vi "lvBuildAll.vi"() -> (0 "error out":errorcluster)   [LabVIEW 2016, in "lvcommonbuild.lvlib"]
uses:
  lvcommonbuild.lvlib
  <vilib>/Wiresmith Technology/LabVIEW CLI/CLI Class/CLI.lvclass
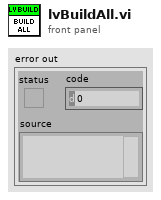
[diagram p1: front panel]
types:
  T1 = typedef "lvcommonbuild.lvlib/ctlTargetInfo.ctl" = cluster{"Target":string, "Build Specs":string[]}
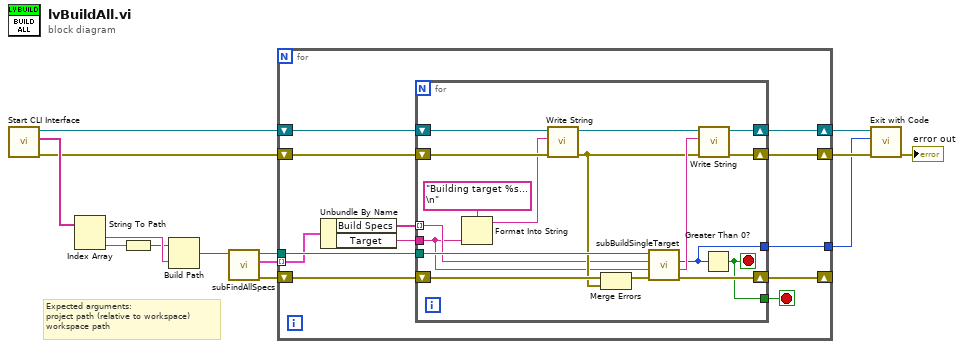
[diagram p0: block diagram]
diagram:
  # "Expected arguments:\nproject path (relative to workspace)\nworkspace path"
  n1 = call <vilib>:"Start CLI Interface.vi"() -> ("error out"=w4:errorcluster, "Custom Parameters"=w14:string[], "CLI out"=w6:refnum<class "CLI.lvclass">)  [unwired: 9 in]
  n2 = Index Array(array=w14) -> (element #1=w12:string, element #2=w1:string)  [unwired: 2 in]
  n3 = String To Path(string=w1) -> (path=w11:path)
  n4 = Build Path(base path=w11, name or relative path=w12) -> (appended path=w10:path)
  n5 = call "subFindAllSpecs.vi"("Project"=w10) -> ("error out"=w9:errorcluster, "Build Specs"=w7:T1[], "dup Project"=w8:path)  [unwired: 8 in]
  n6 = for {
    tunnel: w8 -> [w25]
    tunnel: w7 -> [w19] mode=indexing
    tunnel: [w20] -> w2
    shift-right: [w23] -> w5
    shift-left: w6 -> [w24]
    shift-right: [w21] -> w3
    shift-left: w4 -> [w22]
    shift-right: [w17] -> _
    shift-left: w9 -> [w26]
    stop <- w18 stop-if-true
    n7 = Unbundle By Name(w19) -> ("Build Specs"=w15:string[], "Target"=w16:string)
    n8 = for {
      tunnel: w25 -> [w43]
      shift-right: [w42] -> w23
      shift-left: w24 -> [w36]
      shift-right: [w40] -> w17
      shift-left: w26 -> [w32]
      shift-right: [w39] -> w21
      shift-left: w22 -> [w37]
      tunnel: [w38] -> w20
      tunnel: w15 -> [w29] mode=indexing
      tunnel: w16 -> [w27]
      tunnel: [w28] -> w18
      stop <- w28 stop-if-true
      n9 = Format Into String(format string="Building target %s...\n", w27) -> (resulting string=w33:string)  [unwired: 2 in, 1 out]
      n10 = call <vilib>:"Write String.vi"("error in (no error)"=w37, "Text to Write"=w33, "CLI in"=w36) -> ("error out"=w30:errorcluster, "CLI out"=w35:refnum<class "CLI.lvclass">)  [unwired: 7 in]
      n11 = Merge Errors(w32, w30) -> (w31:errorcluster)
      n12 = call "subBuildSingleTarget.vi"("error in (no error)"=w31, "Target"=w27, "Build Spec"=w29, "Project"=w43) -> ("error out"=w40:errorcluster, "Output Message"=w41:string, "Exit Code (0)"=w38:i32)  [unwired: 5 in]
      n13 = call <vilib>:"Write String.vi"("error in (no error)"=w30, "Text to Write"=w41, "CLI in"=w35) -> ("error out"=w39:errorcluster, "CLI out"=w42:refnum<class "CLI.lvclass">)  [unwired: 7 in]
      n14 = Greater Than 0?(x=w38) -> (x > 0?=w28:bool)
    }
  }
  n15 = call <vilib>:"Exit with Code.vi"("error in (no error)"=w3, "Exit Code (0)"=w2, "CLI in"=w5) -> ("error out"=→"error out":errorcluster)  [unwired: 8 in]
